vi "Result_Test.vi"(8 "error in (no error)":errorcluster caption="entrée d'erreur (pas d'erreur)", 11 "Flash_Jlink en entrée":refnum<class "Check_Func.lvclass">) -> (0 "error out":errorcluster caption="sortie d'erreur", 3 "Flash_Jlink en sortie":refnum<class "Check_Func.lvclass">)   [LabVIEW 2020, in "Library Test.lvlib" / "Check_Func.lvclass"]
uses:
  Check_Func.lvclass
  C:/Users/ngarcin/OneDrive - Altyor/Standard TB/Suite TB45/Class/Test/Test (Default)/Test (Default).lvclass
  Commun VI/TypeDef/Variable Printable.ctl
  Test_Without_Instr/Test_Without_Inst.lvclass
  Commun VI/Library Commun.lvlib
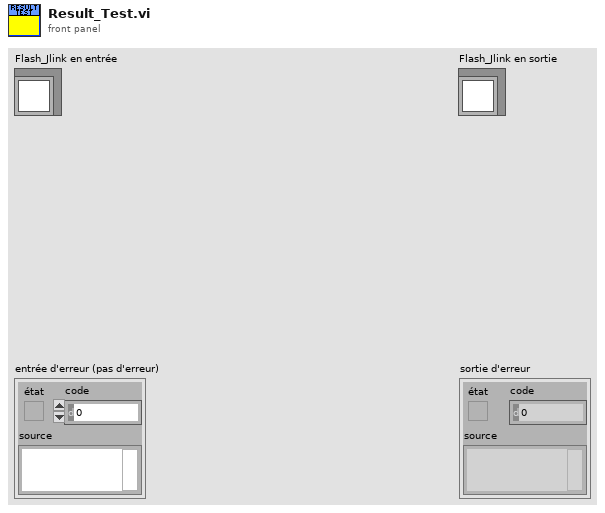
[diagram p1: front panel]
types:
  T1 = enum16{"Get Variable", "Get All Variables", "Set Variable", "Delete Variable", "Delete All Variable"}
  T2 = typedef "Variable Printable.ctl" = string
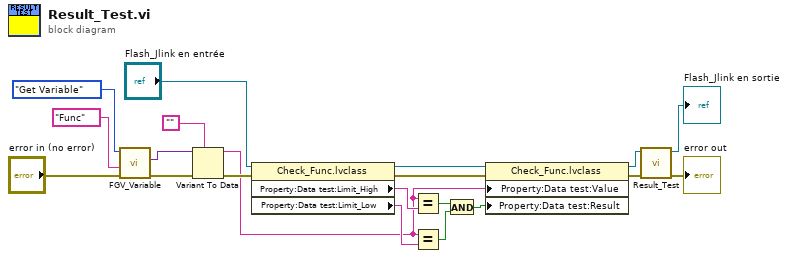
[diagram p0: block diagram]
diagram:
  n1 = call "FGV_Variable.vi"("error in (no error)"="error in (no error)", "Variable"=T2 "Func", "Function"=T1."Get Variable") -> ("error out"=w13:errorcluster, "Data Out"=w12:variant)  [unwired: 6 in, 1 out]
  n2 = Variant To Data(error in=w13, type="", Variant=w12) -> (data=w6:string, error out=w10:errorcluster)
  n3 = property class="Check_Func.lvclass"(reference="Flash_Jlink en entrée", error in=w10) -> (reference out=w1:refnum<class "Check_Func.lvclass">, error out=w9:errorcluster, "Property:Data test:Limit_High"=w8:string, "Property:Data test:Limit_Low"=w7:string)
  n4 = Equal?(x=w6, y=w8) -> (x = y?=w5:bool)
  n5 = Equal?(x=w6, y=w7) -> (x = y?=w4:bool)
  n6 = And(x=w5, y=w4) -> (x .and. y?=w3:bool)
  n7 = property class="Check_Func.lvclass"(reference=w1, error in=w9, "Property:Data test:Value"=w6, "Property:Data test:Result"=w3) -> (reference out=w17:refnum<class "Check_Func.lvclass">, error out=w18:errorcluster)
  n8 = call-parent "Result_Test.vi"("error in (no error)"=w18, "Test_Without_Inst en entrée"=w17) -> ("error out"=→"error out":errorcluster, "Test_Without_Inst en sortie"=→"Flash_Jlink en sortie":refnum<class "Check_Func.lvclass">)  [unwired: 8 in]
